vi "Process Menu Selection.vi"(8 "error in (no error)":errorcluster, 10 "Argument":string, 11 "Menu Ref":refnum<k9>) -> (0 "error out":errorcluster, 3 "State(s) to Enqueue":string)   [LabVIEW 2020, in "MacroAssert.lvlib"]
doc: "Processes any menu selections, enqueuing the next states that need to occur."
uses:
  MacroAssert.lvlib
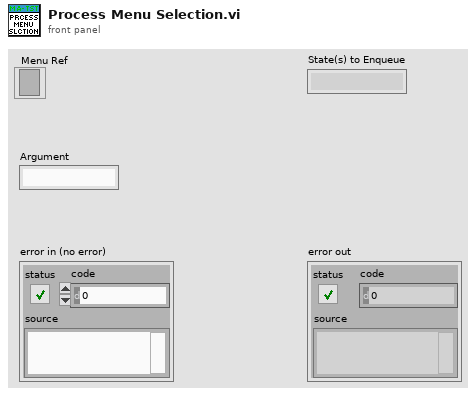
[diagram p1: front panel]
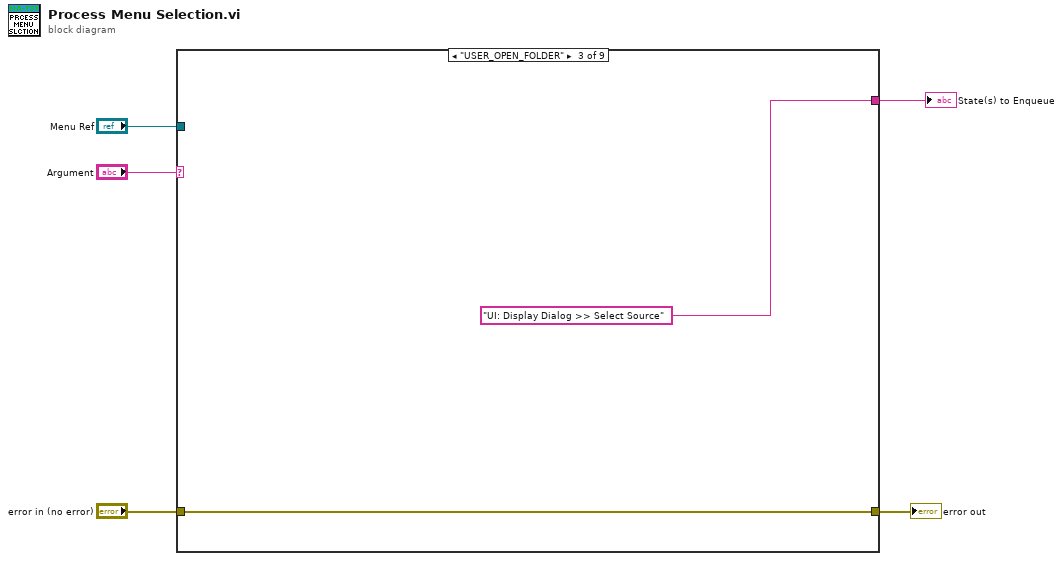
[diagram p0: block diagram]
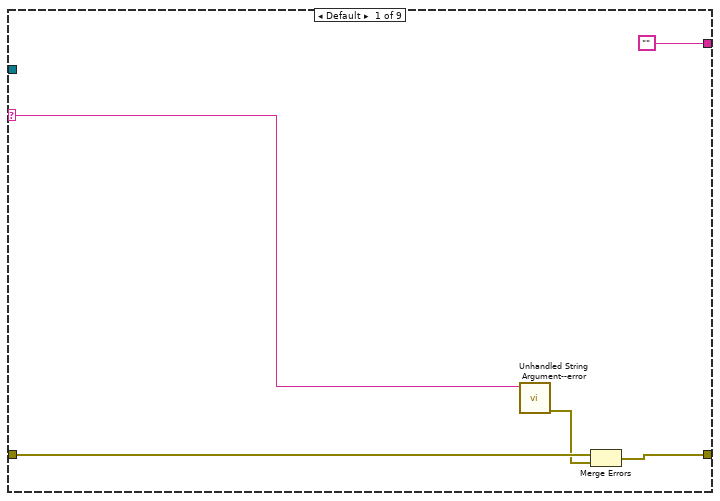
[diagram p2: hidden frame]
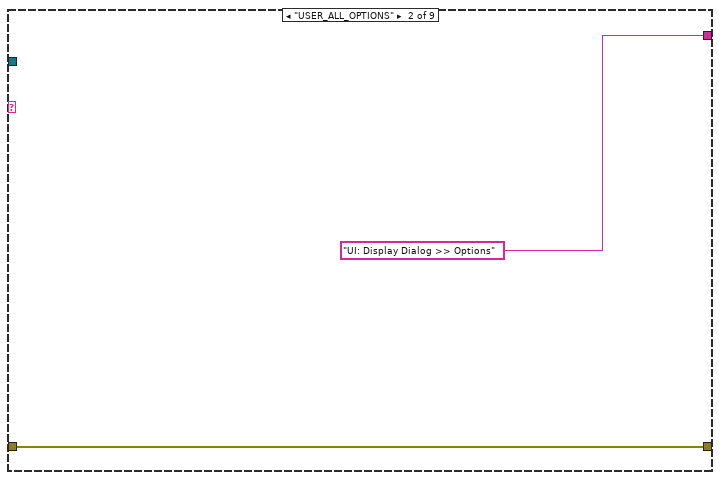
[diagram p3: hidden frame]
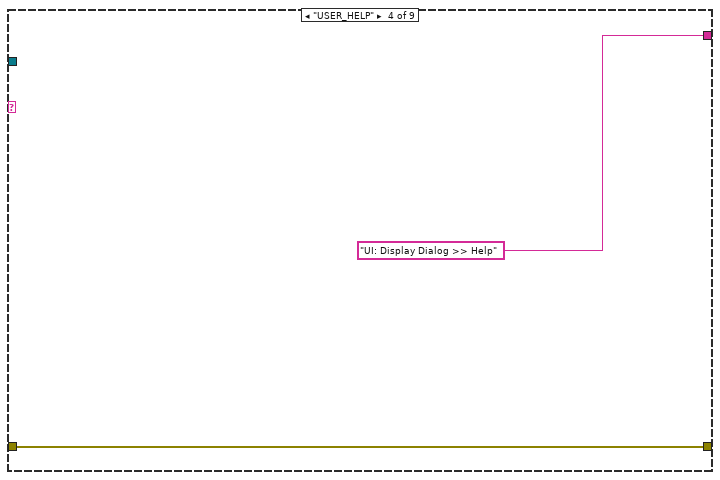
[diagram p4: hidden frame]
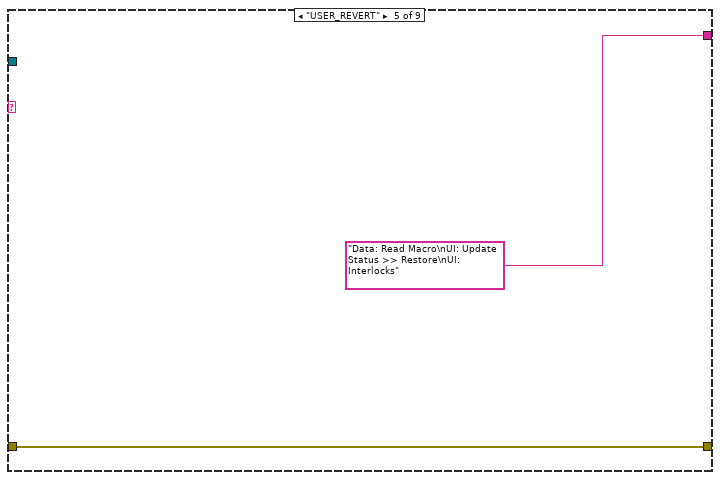
[diagram p5: hidden frame]
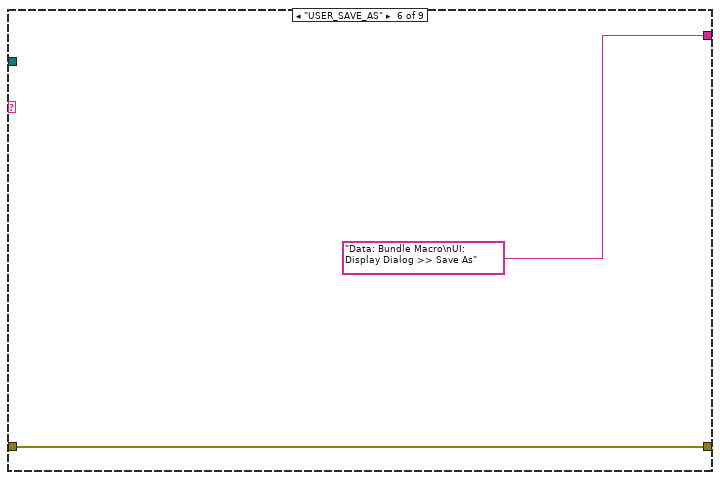
[diagram p6: hidden frame]
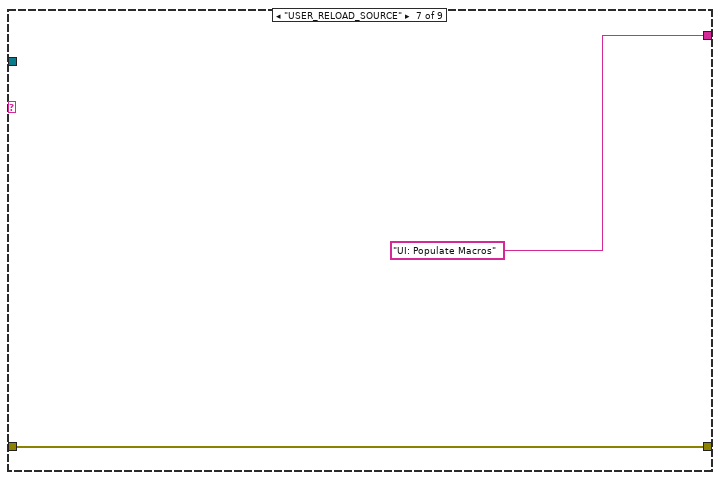
[diagram p7: hidden frame]
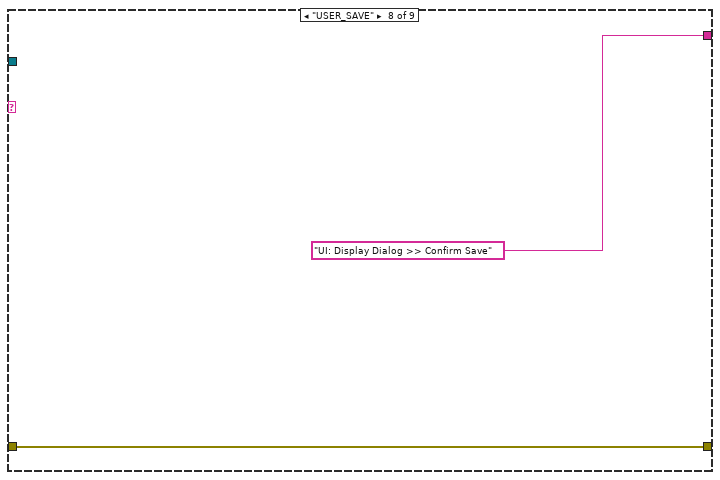
[diagram p8: hidden frame]
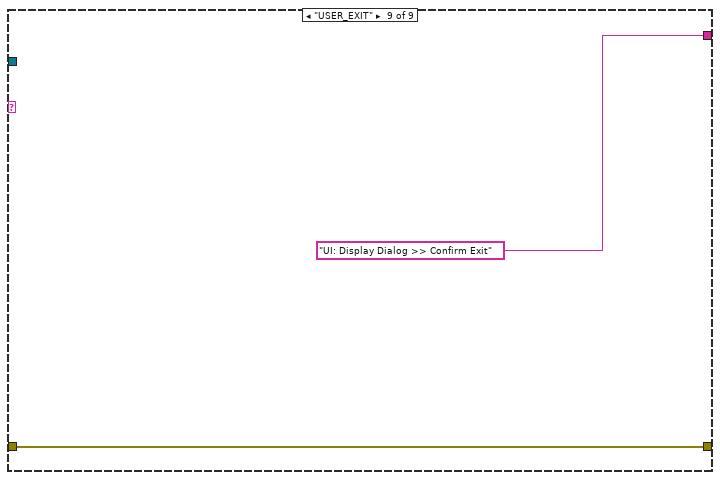
[diagram p9: hidden frame]
diagram:
  n1 = case shown="\"USER_OPEN_FOLDER\"" "Argument" {
    selector: "Argument" -> [w6 _ _ _ _ _ _ _ _]
    tunnel: "error in (no error)" -> [w10 w11 w13 w15 w17 w19 w21 w23 w25]
    tunnel: [w8 w11 w13 w15 w17 w19 w21 w23 w25] -> w3
    tunnel: "Menu Ref" -> [_ _ _ _ _ _ _ _ _]
    tunnel: ["" "UI: Display Dialog >> Options" "UI: Display Dialog >> Select Source" "UI: Display Dialog >> Help" "Data: Read Macro\nUI: Update Status >> Restore\nUI: Interlocks" "Data: Bundle Macro\nUI: Display Dialog >> Save As" "UI: Populate Macros" "UI: Display Dialog >> Confirm Save" "UI: Display Dialog >> Confirm Exit"] -> w1
    frame Default {
      n2 = call "Unhandled String Argument--error.vi"("Argument"=w6) -> ("error out"=w9:errorcluster)  [unwired: 10 in]
      n3 = Merge Errors(w10, w9) -> (w8:errorcluster)
    }
    frame "USER_ALL_OPTIONS" {
    }
    frame "USER_OPEN_FOLDER" {
    }
    frame "USER_HELP" {
    }
    frame "USER_REVERT" {
    }
    frame "USER_SAVE_AS" {
    }
    frame "USER_RELOAD_SOURCE" {
    }
    frame "USER_SAVE" {
    }
    frame "USER_EXIT" {
    }
  }
  "error out" <- w3
  "State(s) to Enqueue" <- w1
